vi "CopyColorImage.vi"(9 "Error in 1":errorcluster, 10 "Image Name":string="untitled", 11 "Image":T1) -> (0 "error out":errorcluster, 1 "error out 2":errorcluster, 2 "Out 2":T1(plugin-control), 3 "Out":T1(plugin-control))   [LabVIEW 2017]
uses:
  <vilib>/vision/Image Controls.llb/IMAQ Image.ctl
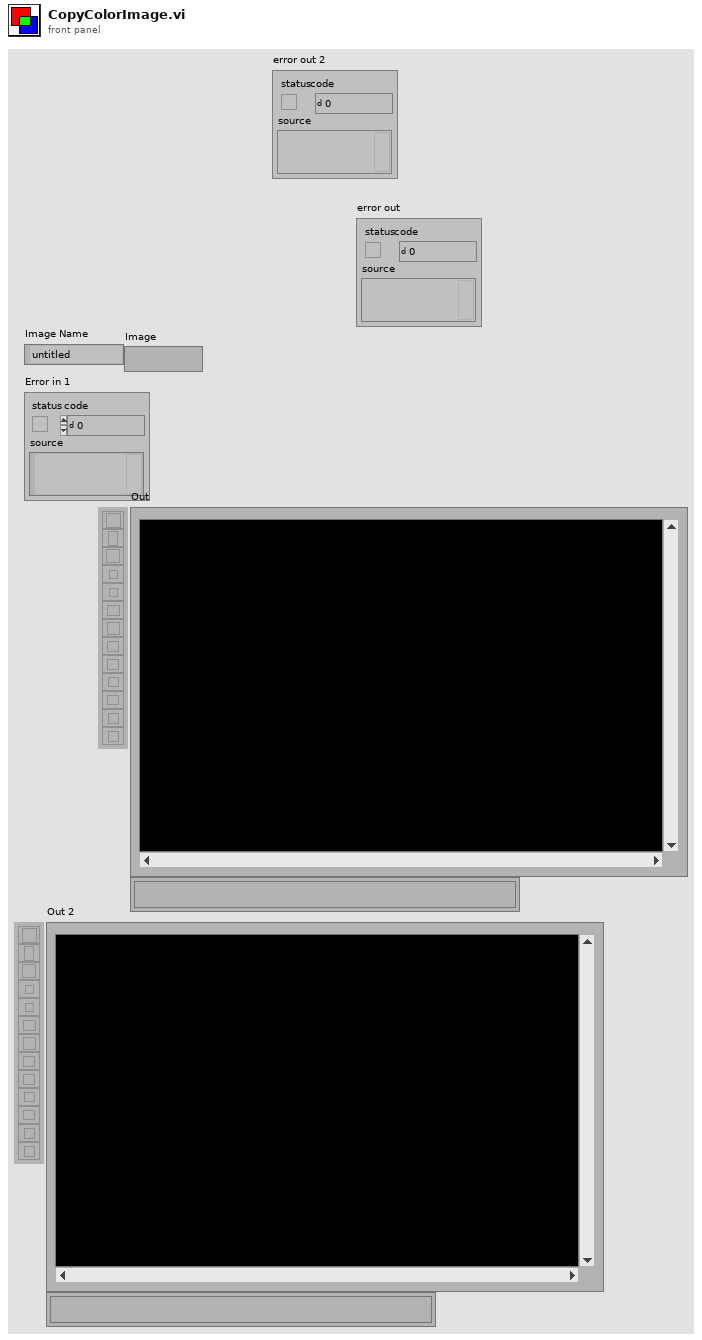
[diagram p1: front panel]
types:
  T1 = typedef "IMAQ Image.ctl" = refnum<image>
  T2 = typedef "Image Type" = u32
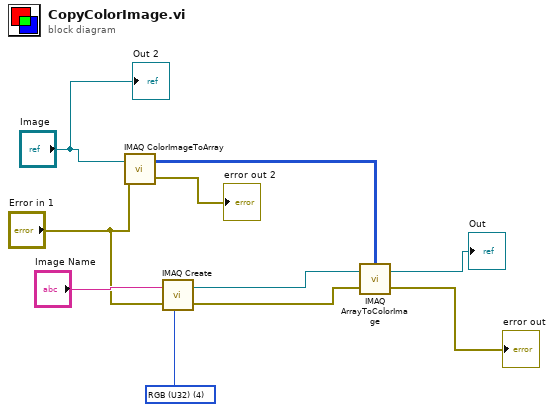
[diagram p0: block diagram]
diagram:
  w2 = T2 4 items=["Grayscale (U8)", "Grayscale (I16)", "Grayscale (SGL)", "Complex (CSG)", "RGB (U32)", "HSL (U32)", "RGB (U64)", "Grayscale (U16)"] ("Image Type")
  n1 = call "IMAQ ColorImageToArray"("Image"="Image", "error in (no error)"="Error in 1") -> ("Image Pixels (U32)"=w7:u32[][], "error out"=→"error out 2":errorcluster)  [unwired: 2 in, 1 out]
  n2 = call "IMAQ Create"("Image Name"="Image Name", "Image Type"=w2, "error in (no error)"="Error in 1") -> ("New Image"=w9:T1, "error out"=w8:errorcluster)  [unwired: 2 in]
  n3 = call "IMAQ ArrayToColorImage"("Image Pixels (U32)"=w7, "Image"=w9, "error in (no error)"=w8) -> ("Image Out"=→"Out":T1, "error out"=→"error out":errorcluster)  [unwired: 2 in]
  "Out 2" <- "Image"
